vi "Main VI FTP FILE MANAGER.vi"() -> ()   [LabVIEW 2012]
doc: "FILE Archive & FTP is a software used to handle the file management of remote field sites using the HTI Data Logger or ATR series acoustic equipment that generates *.RAT and *.ATL files. The software monitors a specific folder on the local machine that the HTI equipment has been set up to move completed files of these types into. All other file types are ignored. The software continues to scan this file until a new file is added to the directory, on the addition of a file the NODE ARCHIVE & FTP software moves the file into an Archive directory (and if specified into a redundant Archive directory) then creates a *.ZIP version of the file and retains a copy of it in the Archive directory as well. All Zip files are then copied to a specified FTP host.\n\nNODE ARCHIVE & FTP will not try and move files for the last five minutes of an hour, or for the first five to ten minutes of the hour (based on CPU time). This is to allow the HTI hardware time to move all files at the top of the hour and avoid conflict. During the rest of the hour the software will continue to scan for new files. At any time a user can force a scan or FTP move by selecting the Manual Force FTP button or the Manual Archive Files button.\n\nNODE ARCHIVE & FTP creates an .INI file and a .CSV file in the programs application directory. The .INI file retains the last values of the file directory and FTP credentials used. The .CSV retains a history of *.ZIP files moved to the FTP and the status of their move, if there were errors or not. NODE ARCHIVE & FTP will continue to try and send the file to the FTP host until that file has completed the process with no errors. DO NOT remove or edit the .CSV file or the software will try and move all files up to the FTP again and will slow down the FTP Host."
uses:
  Controls/FTP Credintials.ctl
  Controls/File Management.ctl
  Controls/File Path directories.ctl
  Controls/Ping address and email notify.ctl
  Controls/PingElements.ctl
  SubVIs/Bini ArchiveAndFtpCluster.ctl
  <vilib>/Utility/sysdir.llb/System Directory Type.ctl
panel:
  in  "SaveConfig":bool
  in  "Settings":bool
  in  "Contacts":bool
  in  "Errors":bool
  in  "SetPingStats":bool
  in  "Addresses to Ping":T1
  in  "File type Cover":bool
  in  "Auto Archive":bool
  in  "Auto FTP":bool
  in  "update extentions":bool
  in  "ShutDown":bool
  in  "FTP Creds":T2={"Host"="", "UserName"="", "PassWord"="", "FTP File Path"="", "Timeout (S)"=0, "ActivePasive"=FALSE, "Binary Ascii"=FALSE, "Remote Port"=21} {"Timeout (S)" min=0 max=300 step=1}
  in  "SITE ID":string="Site Not Configured" caption="Site ID:"
  in  "File Management":T3
  in  "Manual FTP":bool
  out "Archive in progress":bool caption="Archive"
  out "Status FTP move":bool caption="FTP"
  in  "Manual Archive":bool
  in  "File output directories":T4={"Archive Location"=path "", "Archive Location 2"=path "<Not A Path>", "OutPut Path"=path "", "Directory(s) To Scan Files"=[]}
  in  "time date mod":bool
  out "Elapsed Time (H)":dbl caption="Time since Last File \nSize Check (H)" format="%#_3f"
  in  "recipients":string[](array[string])=["nmswyers@gmail.com"] caption="Errors & Warnings Email Recipients"
  out "hours":u8
  out "Email Notification Cluster":T5
  in  "shutting down closeout":bool
  in  "Time DaY":timestamp
  # "D\nI\nR\nE\nC\nT\nO\nR\nY\n\nS\nE\nT"
  # "FILE \n\nHANDLE\n\nMETHODS"
  # "FTP\n\nSETUP"
  # "Passive"
  # "Active"
  # "Binary"
  # "Ascii"
  # "File Handling Method"
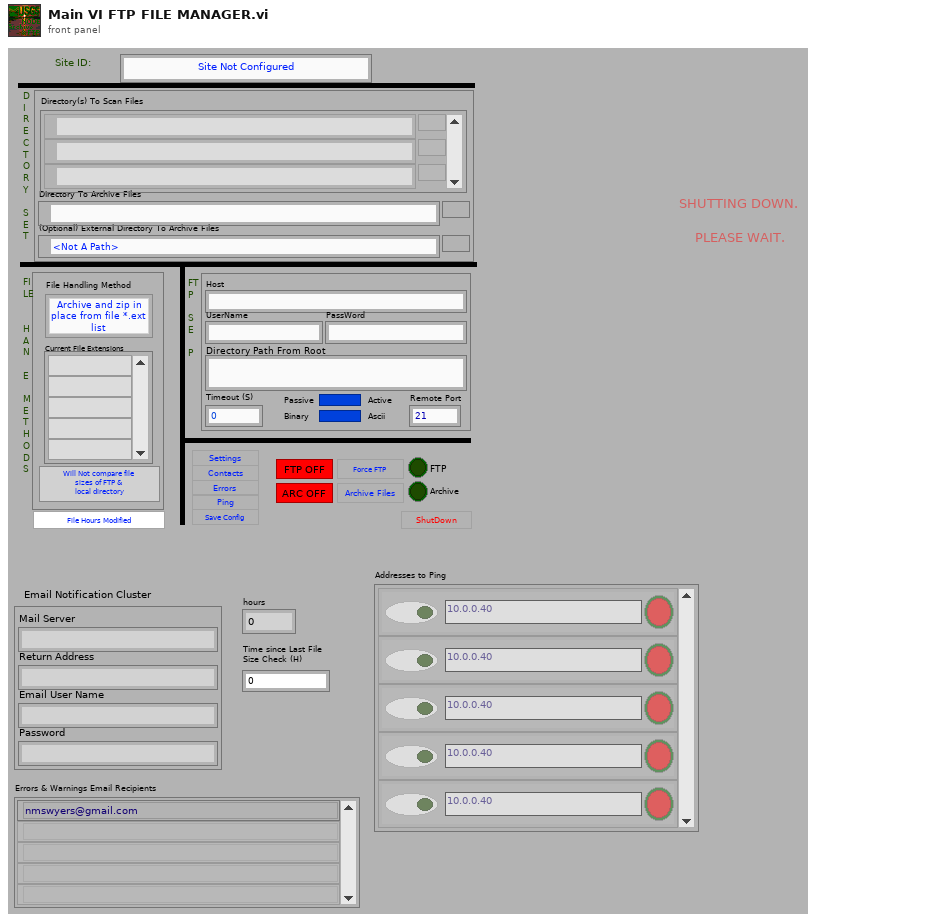
[diagram p1: front panel]
types:
  T1 = typedef "PingElements.ctl" = cluster{"AddressNode 1":string, "Response 1":bool, "Ping on Address 1":bool}[]
  T2 = typedef "FTP Credintials.ctl" = cluster{"Host":string, "UserName":string, "PassWord":string, "FTP File Path":string, "Timeout (S)":i32, "ActivePasive":bool, "Binary Ascii":bool, "Remote Port":u16}
  T3 = typedef "File Management.ctl" = cluster{"Comp File Size":bool, "File Handle Method":enum16{"Archive and zip in place from file *.ext list", "Archive and zip ALL file Types to archive directory", "Archive and zip to archive directory from file *.ext list", "Perform no file management"}, "file extention list":string[]}
  T4 = typedef "File Path directories.ctl" = cluster{"Archive Location":path, "Archive Location 2":path, "OutPut Path":path, "Directory(s) To Scan Files":path[]}
  T5 = typedef "Ping address and email notify.ctl" = cluster{"Mail Server":string, "Return Address":string, "Email User Name":string, "Password":string}
  T6 = enum16{"open", "replace", "create", "open or create", "replace or create", "replace or create with confirmation"}
  T7 = enum8{"Enabled", "Disabled", "Disabled and Grayed Out"}
  T8 = typedef "Bini ArchiveAndFtpCluster.ctl" = cluster{"Site ID":string, "File Management cluster":T3, "time stamp":timestamp, "File output directories":T4, "Auto FTP":bool, "Auto Archive":bool, "FTP CRED Cluster":T2, "hours old date mod(hours)":u8, "Email Notification Cluster":T5, "Email Recipiant List":string[], "Addresses to Ping":T1}
  T9 = enum16{"Archive and zip in place from file *.ext list", "Archive and zip ALL file Types to archive directory", "Archive and zip to archive directory from file *.ext list", "Perform no file management"}
  T10 = enum32{"Invalid", "Standard", "Closed", "Hidden", "Minimized", "Maximized"}
  T11 = cluster{"AddressNode 1":string, "Response 1":bool, "Ping on Address 1":bool}
  T12 = enum32{"invalid app kind", "Development System", "Run Time System", "Student Edition", "Embedded LabVIEW", "Evaluation", "Custom"}
  T13 = typedef "System Directory Type.ctl" = i32
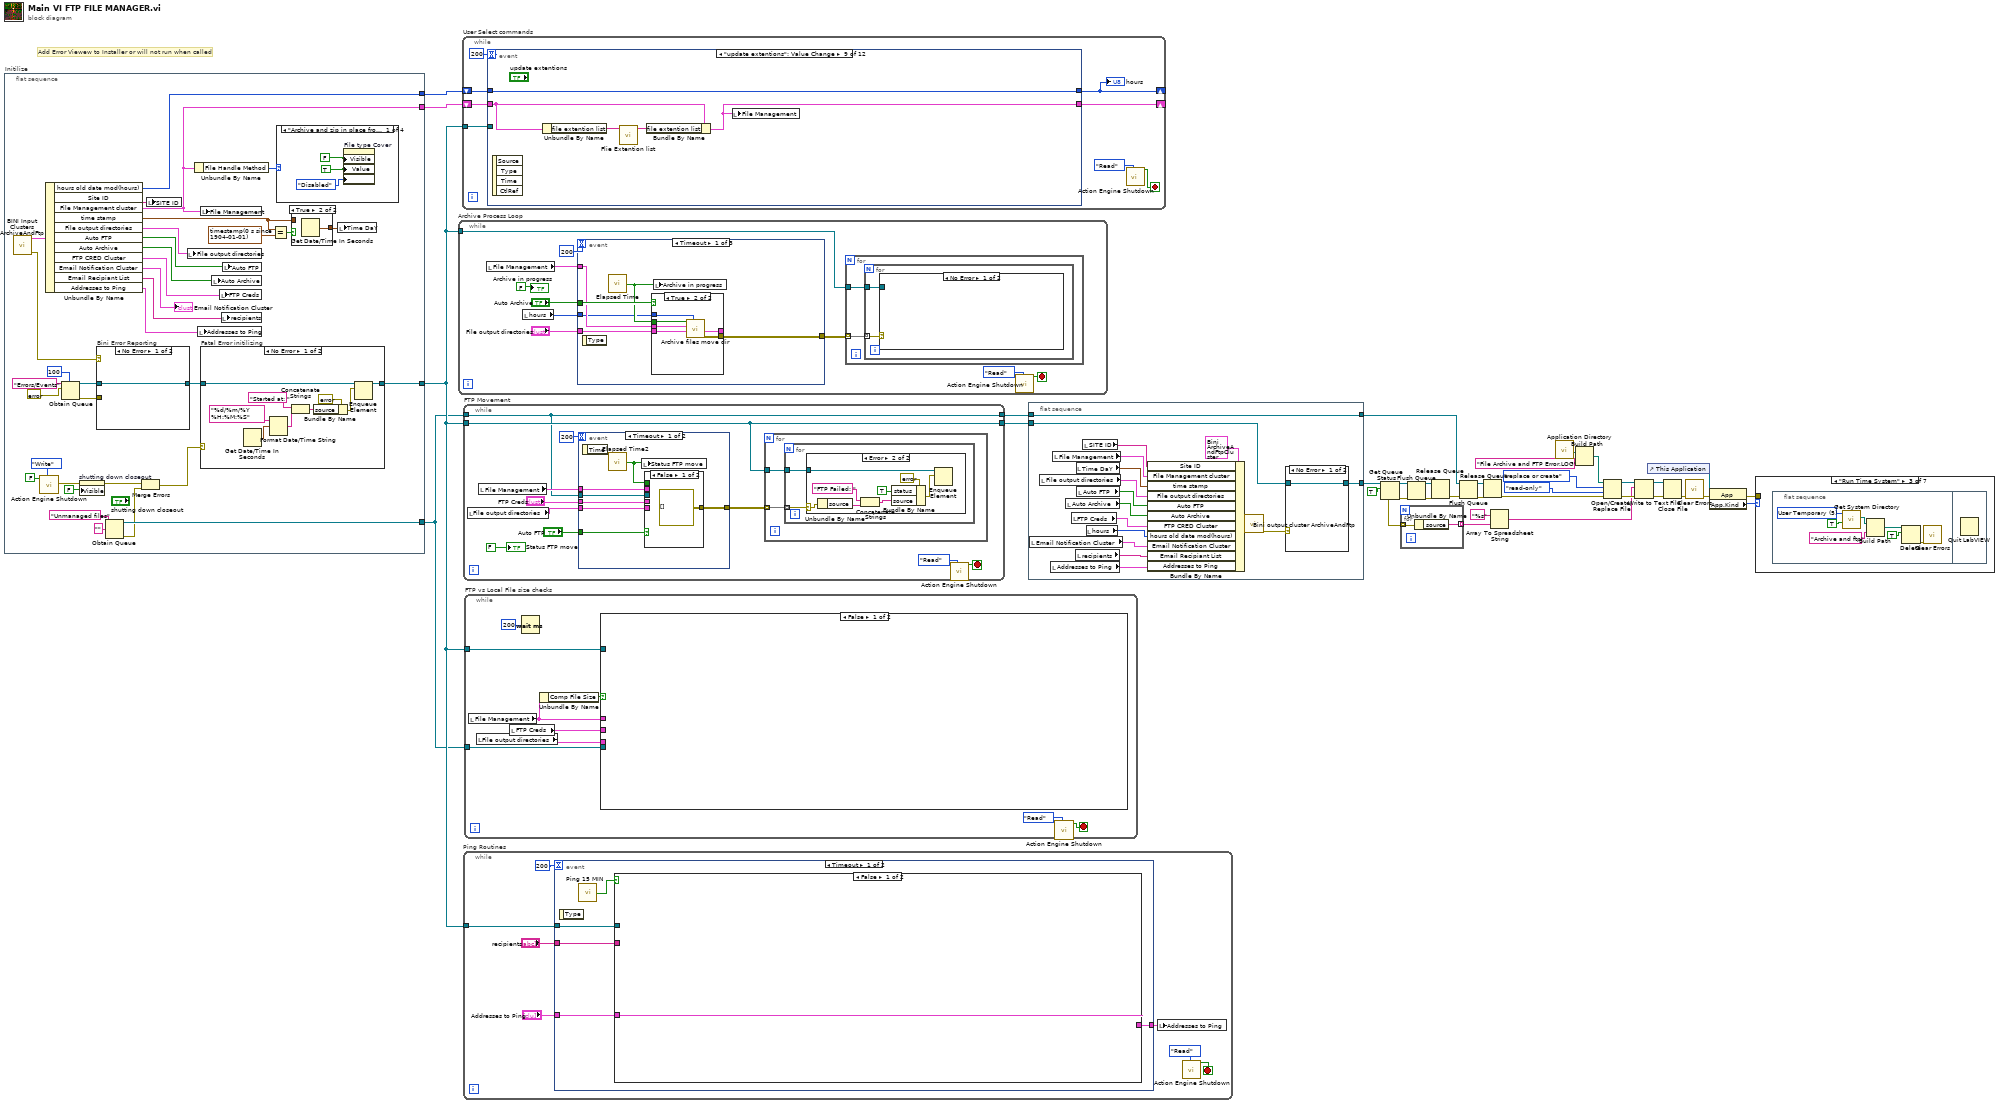
[diagram p0: block diagram]
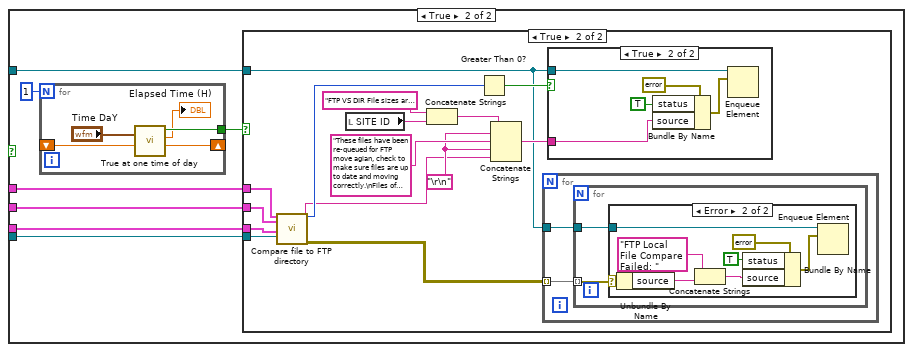
[diagram p2: hidden frame]
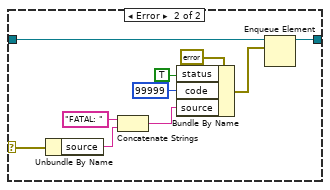
[diagram p7: hidden frame]
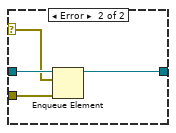
[diagram p8: hidden frame]
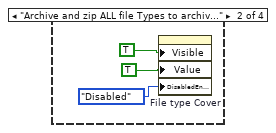
[diagram p9: hidden frame]
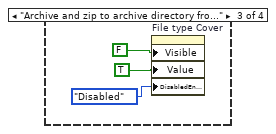
[diagram p10: hidden frame]
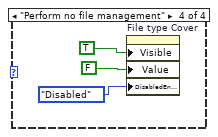
[diagram p11: hidden frame]
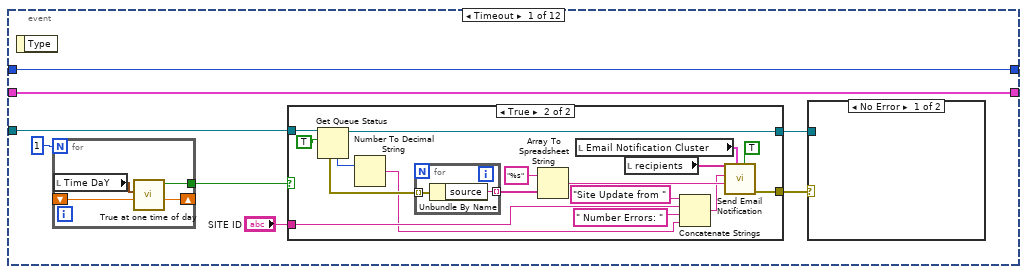
[diagram p12: hidden frame]
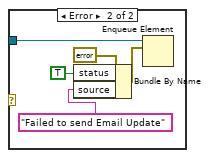
[diagram p13: hidden frame]
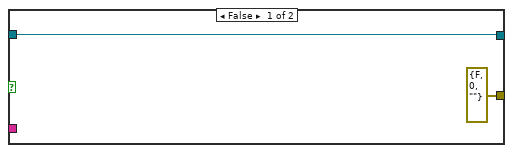
[diagram p14: hidden frame]
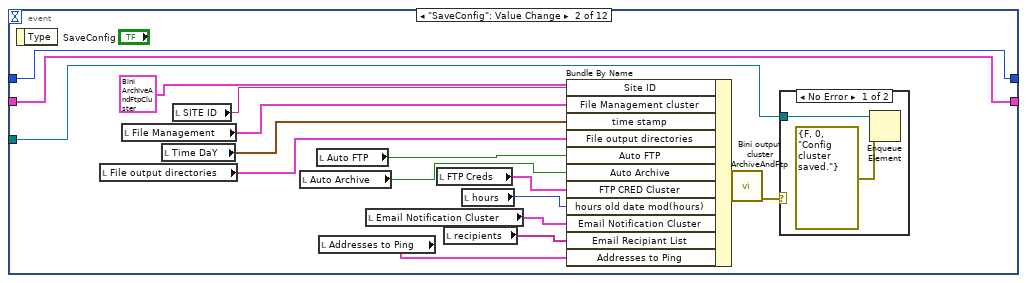
[diagram p15: hidden frame]
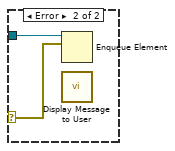
[diagram p16: hidden frame]
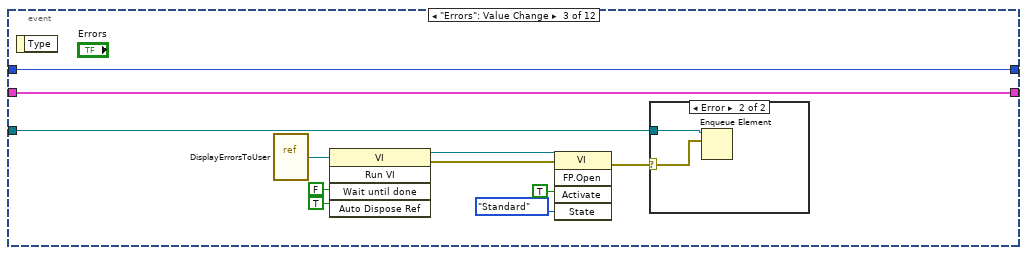
[diagram p17: hidden frame]
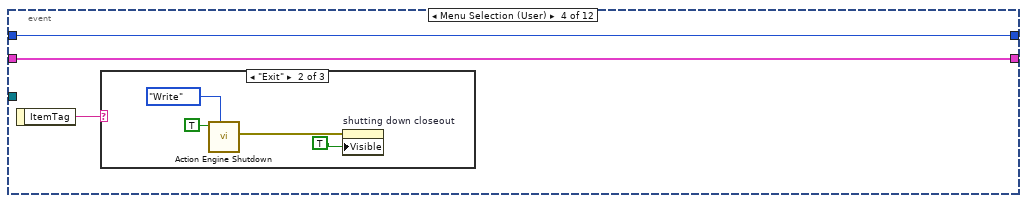
[diagram p19: hidden frame]
diagram:
  # "Add Error Viewew to Installer or will not run when called"
  n1 = flat-sequence "Initilize" {
    tunnel: [w67] -> w29
    tunnel: [w57] -> w32
    tunnel: [w52] -> w31
    tunnel: [w40] -> w30
    frame #0 {
      n2 = call "BINI Input Clusters ArchiveAndFtp.vi"() -> ("Bini Error out"=w47:errorcluster, "Bini Load"=w58:T8)  [unwired: 10 in]
      n3 = call "Action Engine Shutdown.vi"("Shutdown"=enum16{"Write", "Read"}."Write", "Shutdown (True to Shutdown)"=FALSE) -> ("error out"=w63:errorcluster)  [unwired: 8 in, 1 out]
      n4 = Unbundle By Name(w58) -> ("hours old date mod(hours)"=w52:u8, "Site ID"=w56:string, "File Management cluster"=w57:T3, "time stamp"=w36:timestamp, "File output directories"=w55:T4, "Auto FTP"=w54:bool, "Auto Archive"=w53:bool, "FTP CRED Cluster"=w51:T2, "Email Notification Cluster"=→"Email Notification Cluster":T5, "Email Recipiant List"=w49:string[], "Addresses to Ping"=w48:T1)
      n5 = Obtain Queue(max queue size (-1, unlimited)=100, name (unnamed)="Errors/Events", element data type=errorcluster {"status"=FALSE, "code"=0, "source"=""} ("error constant")) -> (queue out=w46:refnum<queue>, error out=w44:errorcluster)  [unwired: 2 in, 1 out]
      n6 = property on="shutting down closeout" class="Bool"(error in=w63, "Visible"=FALSE) -> (error out=w43:errorcluster)  [unwired: 1 in, 1 out]
      n7 = case "Bini Error Reporting" shown="No Error" w47 {
        selector: w47 -> [_ w93]
        tunnel: w46 -> [w91 w95]
        tunnel: [w91 w94] -> w41
        tunnel: w44 -> [_ w92]
        frame No Error {
        }
        frame Error {
          n8 = Enqueue Element(queue=w95, element=w93, error in (no error)=w92) -> (queue out=w94:refnum<queue>)  [unwired: 1 in, 2 out]
        }
      }
      n9 = Obtain Queue(name (unnamed)="Unmanaged files", element data type="" ("name (unnamed)")) -> (queue out=w67:refnum<queue>, error out=w61:errorcluster)  [unwired: 3 in, 1 out]
      n10 = Merge Errors(w43, w61) -> (w42:errorcluster)
      n11 = local write "SITE ID"(w56) -> ()
      n12 = local write "File output directories"(w55) -> ()
      n13 = Unbundle By Name(w57) -> ("File Handle Method"=w62:T9)
      n14 = local write "Addresses to Ping"(w48) -> ()
      n15 = local write "File Management"(w57) -> ()
      n16 = case "Fatal Error initilizing" shown="No Error" w42 {
        selector: w42 -> [_ w84]
        tunnel: w41 -> [w80 w90]
        tunnel: [w79 w89] -> w40
        frame No Error {
          n17 = Get Date/Time In Seconds() -> (seconds since 1Jan1904=w74:timestamp)
          n18 = Format Date/Time String(time format string (%c)="%d/%m/%Y %H:%M:%S", seconds (now)=w74) -> (date/time string=w73:string)  [unwired: 1 in]
          n19 = Concatenate Strings("Started at: " ("string"), w73) -> (w76:string)
          n20 = Bundle By Name(cluster=errorcluster {"status"=FALSE, "code"=0, "source"=""} ("element"), "source"=w76) -> (w77:errorcluster)
          n21 = Enqueue Element(queue=w80, element=w77) -> (queue out=w79:refnum<queue>)  [unwired: 2 in, 2 out]
        }
        frame Error {
          n22 = Unbundle By Name(w84) -> ("source"=w83:string)
          n23 = Concatenate Strings("FATAL: " ("string"), w83) -> (w86:string)
          n24 = Bundle By Name(cluster=errorcluster {"status"=FALSE, "code"=0, "source"=""} ("error constant"), "status"=TRUE, "code"=99999, "source"=w86) -> (w81:errorcluster)
          n25 = Enqueue Element(queue=w90, element=w81) -> (queue out=w89:refnum<queue>)  [unwired: 2 in, 2 out]
        }
      }
      n26 = local write "Auto Archive"(w53) -> ()
      n27 = local write "FTP Creds"(w51) -> ()
      n28 = local write "recipients"(w49) -> ()
      n29 = local write "Auto FTP"(w54) -> ()
      n30 = Equal?(x=w36, y=timestamp(0 s since 1904-01-01)) -> (x = y?=w39:bool)
      n31 = case shown="\"Archive and zip in place from file *.ext list\", Default" w62 {
        frame "Archive and zip in place from file *.ext list", Default {
          n32 = property on="File type Cover" class="Bool (strict)"("Visible"=FALSE, "Value"=TRUE ("File type Cover"), "DisabledEnum"=T7."Disabled" ("Disabled")) -> ()  [unwired: 2 in, 2 out]
        }
        frame "Archive and zip ALL file Types to archive directory" {
          n33 = property on="File type Cover" class="Bool (strict)"("Visible"=TRUE, "Value"=TRUE ("File type Cover"), "DisabledEnum"=T7."Disabled" ("Disabled")) -> ()  [unwired: 2 in, 2 out]
        }
        frame "Archive and zip to archive directory from file *.ext list" {
          n34 = property on="File type Cover" class="Bool (strict)"("Visible"=FALSE, "Value"=TRUE ("File type Cover"), "DisabledEnum"=T7."Disabled" ("Disabled")) -> ()  [unwired: 2 in, 2 out]
        }
        frame "Perform no file management" {
          n35 = property on="File type Cover" class="Bool (strict)"("Visible"=TRUE, "Value"=FALSE ("File type Cover"), "DisabledEnum"=T7."Disabled" ("Disabled")) -> ()  [unwired: 2 in, 2 out]
        }
      }
      n36 = case shown="True" w39 {
        tunnel: [w70 w71] -> w37
        tunnel: w36 -> [w70 _]
        frame False {
        }
        frame True {
          n37 = Get Date/Time In Seconds() -> (seconds since 1Jan1904=w71:timestamp)
        }
      }
      n38 = local write "Time DaY"(w37) -> ()
    }
  }
  n39 = while "Archive Process Loop" {
    tunnel: w30 -> [w109]
    stop <- w113 stop-if-true
    n40 = local read "File Management"() -> (w108:T3)
    n41 = local read "hours"() -> (w110:u8)
    n42 = event shown="[0] Timeout" {
      selector: _ -> [_ _ _]
      dyn-events: _ -> [_ _ _]
      timeout: 200 -> [_ _ _]
      tunnel: [w135 w148 errorcluster[][] [] ("ErrorArray")] -> w112
      tunnel: "File output directories" -> [w130 w147 _]
      tunnel: w108 -> [w133 w145 _]
      tunnel: "Auto Archive" -> [w134 _ _]
      tunnel: w110 -> [w131 w144 _]
      event Timeout {
        n43 = event-data() -> ()  [unwired: 1 in, 1 out]
        n44 = call "Elapsed Time"() -> ("Time has Elapsed"=w132:bool)  [unwired: 12 in, 7 out]
        n45 = case shown="True" w134 {
          tunnel: w130 -> [w137 w143]
          tunnel: [errorcluster[][] [] ("ErrorArray") w142] -> w135
          tunnel: w133 -> [_ w141]
          tunnel: w132 -> [_ w140]
          tunnel: w131 -> [_ w139]
          tunnel: [w137 w138] -> _
          frame False {
          }
          frame True {
            n46 = call "Archive files move dir.vi"("hours old date mod(hours)"=w139, "File path input cluster"=w143, "File Management"=w141, "Timing True to archive"=w140) -> ("ErrorArray"=w142:errorcluster[][], "File path input cluster (out)"=w138:T4)  [unwired: 4 in]
          }
        }
        n47 = local write "Archive in progress"(w132) -> ()
      }
      event "Manual Archive": Value Change {
        w146 = TRUE ("Status File move")
        n48 = event-data() -> ()  [unwired: 1 in, 1 out]
        n49 = local write "Archive in progress"(w146) -> ()
        n50 = call "Archive files move dir.vi"("hours old date mod(hours)"=w144, "File path input cluster"=w147, "File Management"=w145, "Timing True to archive"=w146) -> ("ErrorArray"=w148:errorcluster[][])  [unwired: 4 in, 1 out]
      }
      event Value Change {
        n51 = event-data() -> ("NewVal"=w150:T9)  [unwired: 1 in]
        n52 = case shown="\"Archive and zip ALL file Types to archive directory\"" w150 {
          frame "Archive and zip in place from file *.ext list", Default {
            n53 = property on="File type Cover" class="Bool (strict)"("Visible"=FALSE, "Value"=TRUE ("File type Cover"), "DisabledEnum"=T7."Disabled" ("Disabled")) -> ()  [unwired: 2 in, 2 out]
          }
          frame "Archive and zip ALL file Types to archive directory" {
            n54 = property on="File type Cover" class="Bool (strict)"("Visible"=TRUE, "Value"=TRUE ("File type Cover"), "DisabledEnum"=T7."Disabled" ("Disabled")) -> ()  [unwired: 2 in, 2 out]
          }
          frame "Archive and zip to archive directory from file *.ext list" {
            n55 = property on="File type Cover" class="Bool (strict)"("Visible"=FALSE, "Value"=TRUE ("File type Cover"), "DisabledEnum"=T7."Disabled" ("Disabled")) -> ()  [unwired: 2 in, 2 out]
          }
          frame "Perform no file management" {
            n56 = property on="File type Cover" class="Bool (strict)"("Visible"=TRUE, "Value"=FALSE ("File type Cover"), "DisabledEnum"=T7."Disabled" ("Disabled")) -> ()  [unwired: 2 in, 2 out]
          }
        }
      }
    }
    n57 = for {
      tunnel: w112 -> [w119] mode=indexing
      tunnel: w109 -> [w118]
      n58 = for {
        tunnel: w119 -> [w121] mode=indexing
        tunnel: w118 -> [w120]
        n59 = case shown="No Error" w121 {
          selector: w121 -> [_ w124]
          tunnel: w120 -> [_ w129]
          frame No Error {
          }
          frame Error {
            n60 = Unbundle By Name(w124) -> ("source"=w123:string)
            n61 = Concatenate Strings("Archiving Process: " ("string"), w123) -> (w122:string)
            n62 = Bundle By Name(cluster=errorcluster {"status"=FALSE, "code"=0, "source"=""} ("error constant"), "status"=TRUE, "source"=w122) -> (w127:errorcluster)
            n63 = Enqueue Element(queue=w129, element=w127) -> ()  [unwired: 2 in, 3 out]
          }
        }
      }
    }
    n64 = call "Action Engine Shutdown.vi"("Shutdown"=enum16{"Write", "Read"}."Read") -> ("Shutdown"=w113:bool)  [unwired: 9 in, 1 out]
    "Archive in progress" <- FALSE ("Archive in progress")
  }
  n65 = while "User Select commands" {
    shift-right: [w166] -> _
    shift-left: w31 -> [w167]
    shift-right: [w164] -> _
    shift-left: w32 -> [w165]
    tunnel: w30 -> [w163]
    stop <- w168 stop-if-true
    n66 = event shown="[8] \"update extentions\": Value Change" {
      selector: _ -> [_ _ _ _ _ _ _ _ _ _ _ _]
      dyn-events: _ -> [_ _ _ _ _ _ _ _ _ _ _ _]
      timeout: 200 -> [_ _ _ _ _ _ _ _ _ _ _ _]
      tunnel: w167 -> [w178 w212 w240 w244 w251 w259 w265 w272 w290 w296 w300 w304]
      tunnel: [w178 w212 w240 w244 w251 w259 w265 w271 w290 w296 w300 w304] -> w166
      tunnel: w165 -> [w177 w211 w239 w243 w250 w258 w264 w270 w293 _ w299 w303]
      tunnel: [w177 w211 w239 w243 w250 w258 w264 w270 w291 "File Management" w299 w303] -> w164
      tunnel: w163 -> [w173 w209 w230 _ _ _ _ _ _ _ _ _]
      event Timeout {
        n67 = event-data() -> ()  [unwired: 1 in, 1 out]
        n68 = for {
          N: 1 -> [_]
          tunnel: [w208] -> w176
          shift-right: [w207] -> _
          shift-left: _ -> [w206]
          n69 = local read "Time DaY"() -> (w205:timestamp)
          n70 = call "True at one time of day.vi"("Next start time in"=w206, "Time stamp from INI (only will use time Not date)"=w205) -> ("next start time out"=w207:dbl, "Time has Elapsed"=w208:bool)  [unwired: 6 in, 2 out]
        }
        n71 = case shown="True" w176 {
          tunnel: "SITE ID" -> [_ w190]
          tunnel: w173 -> [w184 w198]
          tunnel: [errorcluster {"status"=FALSE, "code"=0, "source"=""} ("error out") w199] -> w172
          tunnel: [w184 w186] -> w171
          frame False {
          }
          frame True {
            n72 = Get Queue Status(queue=w198, return elements? (F)=TRUE) -> (queue out=w186:refnum<queue>, # elements in queue=w189:i32, elements=w196:errorcluster[])  [unwired: 1 in, 5 out]
            n73 = Number To Decimal String(number=w189) -> (decimal integer string=w187:string)  [unwired: 1 in]
            n74 = for {
              tunnel: w196 -> [w204] mode=indexing
              tunnel: [w203] -> w195 mode=indexing
              n75 = Unbundle By Name(w204) -> ("source"=w203:string)
            }
            n76 = Array To Spreadsheet String(array=w195, 3:"%s" ("format string")) -> (spreadsheet string=w193:string)  [unwired: 1 in]
            n77 = local read "Email Notification Cluster"() -> (w200:T5)
            n78 = local read "recipients"() -> (w202:string[])
            n79 = Concatenate Strings("Site Update from " ("string"), w190, " Number Errors: " ("string"), w187) -> (w192:string)
            n80 = call "Send Email Notification.vi"("Send Email Notification"=TRUE, "Email Notification Cluster (in)"=w200, "message"=w193, "Email Subject"=w192, "recipients"=w202) -> ("error out"=w199:errorcluster)  [unwired: 6 in]
          }
        }
        n81 = case shown="No Error" w172 {
          tunnel: w171 -> [_ w183]
          frame No Error {
          }
          frame Error {
            n82 = Bundle By Name(cluster=errorcluster {"status"=FALSE, "code"=0, "source"=""} ("error constant"), "status"=TRUE, "source"="Failed to send Email Update") -> (w181:errorcluster)
            n83 = Enqueue Element(queue=w183, element=w181) -> ()  [unwired: 2 in, 3 out]
          }
        }
      }
      event "SaveConfig": Value Change {
        n84 = event-data() -> ()  [unwired: 1 in, 1 out]
        n85 = local read "File output directories"() -> (w218:T4)
        n86 = local read "File Management"() -> (w216:T3)
        n87 = local read "Time DaY"() -> (w217:timestamp)
        n88 = local read "SITE ID"() -> (w215:string)
        n89 = local read "Auto Archive"() -> (w220:bool)
        n90 = local read "Auto FTP"() -> (w219:bool)
        n91 = local read "Addresses to Ping"() -> (w225:T1)
        n92 = local read "Email Notification Cluster"() -> (w223:T5)
        n93 = local read "FTP Creds"() -> (w221:T2)
        n94 = local read "recipients"() -> (w224:string[])
        n95 = local read "hours"() -> (w222:u8)
        n96 = Bundle By Name(cluster=T8 {"Site ID"="", "File Management cluster"={"Comp File Size"=FALSE, "File Handle Method"=enum."Archive and zip in place from file *.ext list", "file extention list"=[]}, "time stamp"=timestamp(0 s since 1904-01-01), "File output directories"={"Archive Location"=path "", "Archive Location 2"=path "<Not A Path>", "OutPut Path"=path "", "Directory(s) To Scan Files"=[]}, "Auto FTP"=FALSE, "Auto Archive"=FALSE, "FTP CRED Cluster"={"Host"="", "UserName"="", "PassWord"="", "FTP File Path"="", "Timeout (S)"=60, "ActivePasive"=FALSE, "Binary Ascii"=FALSE, "Remote Port"=0}, "hours old date mod(hours)"=2, "Email Notification Cluster"={"Mail Server"="", "Return Address"="", "Email User Name"="", "Password"=""}, "Email Recipiant List"=[], "Addresses to Ping"=[]} ("Settings To Bini"), "Site ID"=w215, "File Management cluster"=w216, "time stamp"=w217, "File output directories"=w218, "Auto FTP"=w219, "Auto Archive"=w220, "FTP CRED Cluster"=w221, "hours old date mod(hours)"=w222, "Email Notification Cluster"=w223, "Email Recipiant List"=w224, "Addresses to Ping"=w225) -> (w214:T8)
        n97 = call "Bini output cluster ArchiveAndFtp.vi"("Settings To Bini"=w214) -> ("Bini Error out"=w210:errorcluster)  [unwired: 14 in]
        n98 = case shown="No Error" w210 {
          selector: w210 -> [_ w228]
          tunnel: w209 -> [w227 w229]
          frame No Error {
            n99 = Enqueue Element(queue=w227, element=errorcluster {"status"=FALSE, "code"=0, "source"="Config cluster saved."}) -> ()  [unwired: 2 in, 3 out]
          }
          frame Error {
            n100 = Enqueue Element(queue=w229, element=w228) -> ()  [unwired: 2 in, 3 out]
            n101 = call "Display Message to User"() -> ()  [unwired: 10 in, 2 out]
          }
        }
      }
      event "Errors": Value Change {
        n102 = event-data() -> ()  [unwired: 1 in, 1 out]
        n103 = vi-ref "DisplayErrorsToUser.vi"() -> (w238:refnum<vi>)
        n104 = invoke class="VI" method="Run VI"(reference=w238, "Wait until done"=FALSE ("Wait Until Done"), "Auto Dispose Ref"=TRUE ("Auto Dispose Reference")) -> (reference out=w235:refnum<vi>, error out=w234:errorcluster)  [unwired: 2 in, 3 out]
        n105 = invoke class="VI" method="FP.Open"(reference=w235, error in=w234, "Activate"=TRUE ("Activate?"), "State"=T10."Standard") -> (error out=w231:errorcluster)  [unwired: 1 in, 4 out]
        n106 = case shown="Error" w231 {
          selector: w231 -> [_ w241]
          tunnel: w230 -> [_ w242]
          frame No Error {
          }
          frame Error {
            n107 = Enqueue Element(queue=w242, element=w241) -> ()  [unwired: 2 in, 3 out]
          }
        }
      }
      event Menu Selection (User) {
        n108 = event-data() -> ("ItemTag"=w245:string)  [unwired: 1 in]
        n109 = case shown="\"Exit\"" w245 {
          frame "Null", Default {
          }
          frame "Exit" {
            n110 = call "Action Engine Shutdown.vi"("Shutdown"=enum16{"Write", "Read"}."Write", "Shutdown (True to Shutdown)"=TRUE ("Stop Button")) -> ("error out"=w246:errorcluster)  [unwired: 8 in, 1 out]
            n111 = property on="shutting down closeout" class="Bool"(error in=w246, "Visible"=TRUE) -> ()  [unwired: 1 in, 2 out]
          }
          frame "NAF" {
            n112 = call "About.vi"() -> ()  [unwired: 12 in]
          }
        }
      }
      event "ShutDown": Value Change {
        n113 = event-data() -> ()  [unwired: 1 in, 1 out]
        n114 = Two Button Dialog(message="Are you sure you want to shut down the software? This will end all file management of the Archive directories and FTP file movement until the software is restarted.\nIf the Archiving In Progress, or the FTP In Progress is lit the software will shut down as soon as the process is done.", 2:"Shutdown" ("T button name (\"OK\")")) -> (T button?=w254:bool)  [unwired: 1 in]
        n115 = case shown="True" w254 {
          frame False {
          }
          frame True {
            n116 = property on="shutting down closeout" class="Bool"("Visible"=TRUE) -> ()  [unwired: 2 in, 2 out]
            n117 = call "Action Engine Shutdown.vi"("Shutdown"=enum16{"Write", "Read"}."Write", "Shutdown (True to Shutdown)"=TRUE) -> ()  [unwired: 8 in, 2 out]
          }
        }
      }
      event Application Instance Close? {
        w263 = TRUE ("SilentShutdown")
        n118 = event-data() -> ()  [unwired: 1 in, 1 out]
        n119 = call "Action Engine Shutdown.vi"("Shutdown"=enum16{"Write", "Read"}."Write", "Shutdown (True to Shutdown)"=TRUE) -> ()  [unwired: 8 in, 2 out]
        n120 = property on="shutting down closeout" class="Bool"("Visible"=TRUE) -> ()  [unwired: 2 in, 2 out]
        n121 = event-data("SilentShutdown"=w263, "Discard?"=w263) -> ()  [unwired: 1 in, 1 out]
      }
      event Panel Close? {
        n122 = event-data() -> ()  [unwired: 1 in, 1 out]
        n123 = call "Action Engine Shutdown.vi"("Shutdown"=enum16{"Write", "Read"}."Write", "Shutdown (True to Shutdown)"=TRUE) -> ()  [unwired: 8 in, 2 out]
        n124 = property on="shutting down closeout" class="Bool"("Visible"=TRUE) -> ()  [unwired: 2 in, 2 out]
        n125 = event-data("Discard?"=TRUE) -> ()  [unwired: 1 in, 1 out]
      }
      event "time date mod": Value Change {
        n126 = event-data() -> ()  [unwired: 1 in, 1 out]
        n127 = Number To Decimal String(number=w272) -> (decimal integer string=w280:string)  [unwired: 1 in]
        n128 = Concatenate Strings("The Current number of hours that need to passed on a files last modified date before the file will be archived and moved to the ftp server." ("Message"), "\r\n", w280) -> (w278:string)
        n129 = call "Display Message to User2"("Message"=w278) -> ("error out"=w275:errorcluster, "Change Value"=w276:bool)  [unwired: 9 in]
        n130 = call "Prompt User for Input2"("Enable"=w276, "error in (no error)"=w275) -> ("(Hours)"=w274:dbl, "OK"=w273:bool, "error out"=w281:errorcluster)  [unwired: 15 in]
        n131 = case shown="No Error" w281 {
          tunnel: w273 -> [w285 _]
          tunnel: w274 -> [w284 _]
          tunnel: [w283 w289] -> w271
          tunnel: w272 -> [w282 w289]
          frame No Error {
            n132 = case shown="True" w285 {
              tunnel: w284 -> [_ w288]
              tunnel: w282 -> [w286 _]
              tunnel: [w286 w287] -> w283
              frame False {
              }
              frame True {
                n133 = To Unsigned Byte Integer(number=w288) -> (unsigned 8bit integer=w287:u8)
              }
            }
          }
          frame Error {
          }
        }
      }
      event "update extentions": Value Change {
        n134 = event-data() -> ()  [unwired: 1 in, 4 out]
        n135 = Unbundle By Name(w293) -> ("file extention list"=w292:string[])
        n136 = call "Flie Extention list.vi"("file extention list IN"=w292) -> ("File extention list (out)"=w294:string[])  [unwired: 10 in]
        n137 = Bundle By Name(cluster=w293, "file extention list"=w294) -> (w291:T3)
        n138 = local write "File Management"(w291) -> ()
      }
      event Value Change {
        n139 = event-data() -> ()  [unwired: 1 in, 4 out]
        n140 = local write "File Management"("File Management") -> ()
      }
      event "Contacts": Value Change {
        n141 = event-data() -> ()  [unwired: 1 in, 1 out]
        n142 = local read "recipients"() -> (w298:string[])
        n143 = call "SetContactList.vi"("recipients IN"=w298) -> ("recipients OUT"=w297:string[])  [unwired: 10 in]
        n144 = local write "recipients"(w297) -> ()
      }
      event "Settings": Value Change {
        n145 = event-data() -> ()  [unwired: 1 in, 1 out]
        n146 = local read "Email Notification Cluster"() -> (w302:T5)
        n147 = call "GeneralSettingsConfigure.vi"("Email Notification Cluster in"=w302) -> ("Email Notification Cluster out"=w301:T5)  [unwired: 10 in]
        n148 = local write "Email Notification Cluster"(w301) -> ()
      }
    }
    "hours" <- w166
    n149 = call "Action Engine Shutdown.vi"("Shutdown"=enum16{"Write", "Read"}."Read") -> ("Shutdown"=w168:bool)  [unwired: 9 in, 1 out]
  }
  n150 = while "Ping Routines" {
    tunnel: w30 -> [w307]
    stop <- w308 stop-if-true
    n151 = event shown="[0] Timeout" {
      selector: _ -> [_ _]
      dyn-events: _ -> [_ _]
      timeout: 200 -> [_ _]
      tunnel: "recipients" -> [w315 _]
      tunnel: "Addresses to Ping" -> [w314 w374]
      tunnel: w307 -> [w313 _]
      tunnel: [w312 w373] -> w306
      event Timeout {
        n152 = event-data() -> ()  [unwired: 1 in, 1 out]
        n153 = call "Ping 15 MIN"() -> ("Time has Elapsed"=w316:bool)  [unwired: 12 in, 7 out]
        n154 = case shown="False" w316 {
          tunnel: w315 -> [_ w321]
          tunnel: w314 -> [w317 w320]
          tunnel: w313 -> [_ w319]
          tunnel: [w317 w318] -> w312
          frame False {
          }
          frame True {
            n155 = for {
              tunnel: w321 -> [w329]
              tunnel: w320 -> [w324] mode=indexing
              tunnel: w319 -> [w323]
              tunnel: [w322] -> w318 mode=indexing
              stop <- w326 stop-if-true
              n156 = Unbundle By Name(w324) -> ("AddressNode 1"=w325:string, "Ping on Address 1"=w328:bool)
              n157 = case shown="True" w328 {
                tunnel: w325 -> [_ w337]
                tunnel: w329 -> [_ w340]
                tunnel: w324 -> [w332 w338]
                tunnel: w323 -> [_ w334]
                tunnel: [w330 w333] -> w322
                frame False {
                  n158 = Bundle By Name(cluster=w332, "Response 1"=FALSE) -> (w330:T11)
                }
                frame True {
                  n159 = call "Online Status through Ping.vi"("AddressToPing"=w337, "Ping Method"=enum16{"LongPing", "NormalPing", "FastPing"}."FastPing") -> ("Connection?"=w339:bool, "error out"=w335:errorcluster)  [unwired: 9 in, 3 out]
                  n160 = case shown="No Error" w335 {
                    selector: w335 -> [_ w365]
                    tunnel: w340 -> [w346 _]
                    tunnel: w339 -> [w345 _]
                    tunnel: w338 -> [w344 w368]
                    tunnel: w337 -> [w343 w362]
                    tunnel: w334 -> [w342 w372]
                    tunnel: [w341 w366] -> w333
                    frame No Error {
                      n161 = case shown="False" w345 {
                        tunnel: w346 -> [_ _]
                        tunnel: w343 -> [w347 _]
                        tunnel: w344 -> [w356 w359]
                        tunnel: w342 -> [w353 _]
                        tunnel: [w355 w357] -> w341
                        frame False {
                          n162 = Bundle By Name(cluster=w356, "Response 1"=FALSE) -> (w355:T11)
                          n163 = Concatenate Strings("Unable to Ping: " ("string"), w347) -> (w349:string)
                          n164 = Bundle By Name(cluster=errorcluster {"status"=FALSE, "code"=0, "source"=""} ("error constant"), "status"=FALSE, "source"=w349) -> (w351:errorcluster)
                          n165 = Enqueue Element(queue=w353, element=w351) -> ()  [unwired: 2 in, 3 out]
                        }
                        frame True {
                          n166 = Bundle By Name(cluster=w359, "Response 1"=TRUE) -> (w357:T11)
                        }
                      }
                    }
                    frame Error {
                      n167 = Unbundle By Name(w365) -> ("source"=w360:string)
                      n168 = Bundle By Name(cluster=w368, "Response 1"=FALSE) -> (w366:T11)
                      n169 = Concatenate Strings("Ping Request Failed on IP: " ("string"), w362, " : " ("string"), w360) -> (w364:string)
                      n170 = Bundle By Name(cluster=errorcluster {"status"=FALSE, "code"=0, "source"=""} ("error constant"), "status"=TRUE, "source"=w364) -> (w370:errorcluster)
                      n171 = Enqueue Element(queue=w372, element=w370) -> ()  [unwired: 2 in, 3 out]
                    }
                  }
                }
              }
              n172 = call "Action Engine Shutdown.vi"("Shutdown"=enum16{"Write", "Read"}."Read") -> ("Shutdown"=w326:bool)  [unwired: 9 in, 1 out]
            }
          }
        }
      }
      event "SetPingStats": Value Change {
        n173 = event-data() -> ()  [unwired: 1 in, 1 out]
        n174 = call "SetPingAddresses.vi"("Addresses to Ping(in)"=w374) -> ("Addresses to Ping(out)"=w373:T1)  [unwired: 10 in]
      }
    }
    n175 = local write "Addresses to Ping"(w306) -> ()
    n176 = call "Action Engine Shutdown.vi"("Shutdown"=enum16{"Write", "Read"}."Read") -> ("Shutdown"=w308:bool)  [unwired: 9 in, 1 out]
  }
  n177 = while "FTP Movement" {
    tunnel: w29 -> [w376]
    tunnel: w30 -> [w377]
    tunnel: [w377] -> w28
    tunnel: [w376] -> w7
    stop <- w379 stop-if-true
    n178 = local read "File output directories"() -> (w383:T4)
    n179 = local read "File Management"() -> (w381:T3)
    n180 = event shown="[0] Timeout" {
      selector: _ -> [_ _]
      dyn-events: _ -> [_ _]
      timeout: 200 -> [_ _]
      tunnel: w376 -> [w404 w415]
      tunnel: [w403 w416] -> w375
      tunnel: "FTP Creds" -> [w402 w414]
      tunnel: w383 -> [w400 w412]
      tunnel: w381 -> [w401 w413]
      tunnel: "Auto FTP" -> [w399 _]
      event Timeout {
        n181 = event-data() -> ()  [unwired: 1 in, 1 out]
        n182 = call "Elapsed Time2"() -> ("Time has Elapsed"=w398:bool)  [unwired: 12 in, 7 out]
        n183 = local write "Status FTP move"(w398) -> ()
        n184 = case shown="False" w399 {
          tunnel: w398 -> [_ w411]
          tunnel: [errorcluster[][] [] ("ErrorArray") w410] -> w403
          tunnel: w404 -> [_ w409]
          tunnel: w401 -> [_ w408]
          tunnel: w402 -> [_ w407]
          tunnel: w400 -> [_ w406]
          frame False {
          }
          frame True {
            n185 = call "FTP Move files.vi"("File Management"=w408, "Unmanaged Files Queue"=w409, "FTP Creds"=w407, "File output directories"=w406, "Timing true or false to zip files"=w411) -> ("ErrorArray"=w410:errorcluster[][])  [unwired: 13 in, 1 out]
          }
        }
      }
      event "Manual FTP": Value Change {
        n186 = event-data() -> ()  [unwired: 1 in, 1 out]
        n187 = local write "Status FTP move"(TRUE ("Status FTP move")) -> ()
        n188 = call "FTP Move files.vi"("File Management"=w413, "Unmanaged Files Queue"=w415, "FTP Creds"=w414, "File output directories"=w412, "Timing true or false to zip files"=TRUE) -> ("ErrorArray"=w416:errorcluster[][])  [unwired: 13 in, 1 out]
      }
    }
    n189 = for {
      tunnel: w377 -> [w387]
      tunnel: w375 -> [w386] mode=indexing
      n190 = for {
        tunnel: w387 -> [w389]
        tunnel: w386 -> [w388] mode=indexing
        n191 = case shown="Error" w388 {
          selector: w388 -> [_ w393]
          tunnel: w389 -> [_ w397]
          frame No Error {
          }
          frame Error {
            n192 = Unbundle By Name(w393) -> ("source"=w392:string)
            n193 = Concatenate Strings("FTP Failed: " ("string"), w392) -> (w391:string)
            n194 = Bundle By Name(cluster=errorcluster {"status"=FALSE, "code"=0, "source"=""} ("error constant"), "status"=TRUE, "source"=w391) -> (w395:errorcluster)
            n195 = Enqueue Element(queue=w397, element=w395) -> ()  [unwired: 2 in, 3 out]
          }
        }
      }
    }
    n196 = call "Action Engine Shutdown.vi"("Shutdown"=enum16{"Write", "Read"}."Read") -> ("Shutdown"=w379:bool)  [unwired: 9 in, 1 out]
    "Status FTP move" <- FALSE ("Status FTP move")
  }
  n197 = while "FTP vs Local File size checks" {
    tunnel: w30 -> [w422]
    tunnel: w29 -> [w425]
    stop <- w420 stop-if-true
    n198 = local read "File Management"() -> (w427:T3)
    n199 = local read "File output directories"() -> (w424:T4)
    n200 = local read "FTP Creds"() -> (w423:T2)
    n201 = Wait (ms)(milliseconds to wait=u32 200) -> ()  [unwired: 1 out]
    n202 = Unbundle By Name(w427) -> ("Comp File Size"=w426:bool)
    n203 = case shown="False" w426 {
      tunnel: w427 -> [_ w432]
      tunnel: w425 -> [_ w431]
      tunnel: w424 -> [_ w430]
      tunnel: w423 -> [_ w429]
      tunnel: w422 -> [_ w428]
      frame False {
      }
      frame True {
        n204 = for {
          N: 1 -> [_]
          tunnel: [w438] -> w434
          shift-right: [w436] -> _
          shift-left: _ -> [w435]
          n205 = call "True at one time of day.vi"("Next start time in"=w435, "Time stamp from INI (only will use time Not date)"="Time DaY") -> ("next start time out"=w436:dbl, "Time Until Next Scan (H)"=→"Elapsed Time (H)":dbl, "Time has Elapsed"=w438:bool)  [unwired: 6 in, 1 out]
        }
        n206 = case shown="True" w434 {
          tunnel: w432 -> [_ w447]
          tunnel: w431 -> [_ w446]
          tunnel: w430 -> [_ w445]
          tunnel: w429 -> [_ w444]
          tunnel: w428 -> [_ w441]
          frame False {
          }
          frame True {
            w452 = "\r\n"
            n207 = call "Compare file to FTP directory.vi"("File Management"=w447, "FTP Creds"=w444, "File output directories"=w445, "Unmanaged Files Queue"=w446) -> ("number of unmached files"=w449:i32, "unmatched file names"=w448:string, "ErrorArray"=w440:errorcluster[][])  [unwired: 12 in, 1 out]
            n208 = local read "SITE ID"() -> (w450:string)
            n209 = Concatenate Strings("FTP VS DIR File sizes are different: " ("string"), w450) -> (w451:string)
            n210 = Greater Than 0?(x=w449) -> (x > 0?=w443:bool)
            n211 = Concatenate Strings(w451, w452, "These files have been re-queued for FTP move agian, check to make sure files are up to date and moving correctly.\nFiles of issue are listed below.\n\nLIST:" ("string"), w452, w448) -> (w442:string)
            n212 = for {
              tunnel: w441 -> [w456]
              tunnel: w440 -> [w455] mode=indexing
              n213 = for {
                tunnel: w456 -> [w458]
                tunnel: w455 -> [w457] mode=indexing
                n214 = case shown="Error" w457 {
                  selector: w457 -> [_ w461]
                  tunnel: w458 -> [_ w466]
                  frame No Error {
                  }
                  frame Error {
                    n215 = Unbundle By Name(w461) -> ("source"=w460:string)
                    n216 = Concatenate Strings("FTP Local File Compare Failed: " ("string"), w460) -> (w462:string)
                    n217 = Bundle By Name(cluster=errorcluster {"status"=FALSE, "code"=0, "source"=""} ("error constant"), "status"=TRUE, "source"=w462) -> (w464:errorcluster)
                    n218 = Enqueue Element(queue=w466, element=w464) -> ()  [unwired: 2 in, 3 out]
                  }
                }
              }
            }
            n219 = case shown="True" w443 {
              tunnel: w441 -> [_ w471]
              tunnel: w442 -> [_ w467]
              frame False {
              }
              frame True {
                n220 = Bundle By Name(cluster=errorcluster {"status"=FALSE, "code"=0, "source"=""} ("error constant"), "status"=TRUE, "source"=w467) -> (w469:errorcluster)
                n221 = Enqueue Element(queue=w471, element=w469) -> ()  [unwired: 2 in, 3 out]
              }
            }
          }
        }
      }
    }
    n222 = call "Action Engine Shutdown.vi"("Shutdown"=enum16{"Write", "Read"}."Read") -> ("Shutdown"=w420:bool)  [unwired: 9 in, 1 out]
  }
  n223 = flat-sequence {
    tunnel: w28 -> [w474]
    tunnel: [w473] -> w27
    tunnel: w7 -> [w472]
    tunnel: [w472] -> w4
    frame #0 {
      n224 = local read "Email Notification Cluster"() -> (w478:T5)
      n225 = local read "File output directories"() -> (w483:T4)
      n226 = local read "Addresses to Ping"() -> (w476:T1)
      n227 = local read "File Management"() -> (w485:T3)
      n228 = local read "Auto Archive"() -> (w481:bool)
      n229 = local read "FTP Creds"() -> (w480:T2)
      n230 = local read "recipients"() -> (w477:string[])
      n231 = local read "Time DaY"() -> (w484:timestamp)
      n232 = local read "Auto FTP"() -> (w482:bool)
      n233 = local read "SITE ID"() -> (w486:string)
      n234 = local read "hours"() -> (w479:u8)
      n235 = Bundle By Name(cluster=T8 {"Site ID"="", "File Management cluster"={"Comp File Size"=FALSE, "File Handle Method"=enum."Archive and zip in place from file *.ext list", "file extention list"=[]}, "time stamp"=timestamp(0 s since 1904-01-01), "File output directories"={"Archive Location"=path "", "Archive Location 2"=path "<Not A Path>", "OutPut Path"=path "", "Directory(s) To Scan Files"=[]}, "Auto FTP"=FALSE, "Auto Archive"=FALSE, "FTP CRED Cluster"={"Host"="", "UserName"="", "PassWord"="", "FTP File Path"="", "Timeout (S)"=60, "ActivePasive"=FALSE, "Binary Ascii"=FALSE, "Remote Port"=0}, "hours old date mod(hours)"=2, "Email Notification Cluster"={"Mail Server"="", "Return Address"="", "Email User Name"="", "Password"=""}, "Email Recipiant List"=[], "Addresses to Ping"=[]} ("Settings To Bini"), "Site ID"=w486, "File Management cluster"=w485, "time stamp"=w484, "File output directories"=w483, "Auto FTP"=w482, "Auto Archive"=w481, "FTP CRED Cluster"=w480, "hours old date mod(hours)"=w479, "Email Notification Cluster"=w478, "Email Recipiant List"=w477, "Addresses to Ping"=w476) -> (w487:T8)
      n236 = call "Bini output cluster ArchiveAndFtp.vi"("Settings To Bini"=w487) -> ("Bini Error out"=w475:errorcluster)  [unwired: 14 in]
      n237 = case shown="No Error" w475 {
        selector: w475 -> [_ w491]
        tunnel: w474 -> [w489 w492]
        tunnel: [w489 w490] -> w473
        frame No Error {
        }
        frame Error {
          n238 = Enqueue Element(queue=w492, element=w491) -> (queue out=w490:refnum<queue>)  [unwired: 2 in, 2 out]
        }
      }
    }
  }
  n239 = Get Queue Status(queue=w27, return elements? (F)=TRUE) -> (queue out=w20:refnum<queue>, error out=w19:errorcluster, elements=w25:errorcluster[])  [unwired: 1 in, 5 out]
  n240 = for {
    tunnel: w25 -> [w494] mode=indexing
    tunnel: [w493] -> w24 mode=indexing
    n241 = Unbundle By Name(w494) -> ("source"=w493:string)
  }
  n242 = Flush Queue(queue=w20, error in (no error)=w19) -> (queue out=w22:refnum<queue>, error out=w21:errorcluster)  [unwired: 1 out]
  n243 = Release Queue(queue=w22, error in (no error)=w21) -> (error out=w5:errorcluster)  [unwired: 1 in, 2 out]
  n244 = Flush Queue(queue=w4, error in (no error)=w5) -> (queue out=w6:refnum<queue>, error out=w3:errorcluster)  [unwired: 1 out]
  n245 = Release Queue(queue=w6, error in (no error)=w3) -> (error out=w2:errorcluster)  [unwired: 1 in, 2 out]
  n246 = Array To Spreadsheet String(array=w24, 3:"%s" ("format string")) -> (spreadsheet string=w8:string)  [unwired: 1 in]
  n247 = call <vilib>:"Application Directory.vi"() -> ("Application Directory"=w17:path)
  n248 = Build Path(base path=w17, name or relative path="File Archive and FTP Error.LOG") -> (appended path=w14:path)
  n249 = Open/Create/Replace File(file path (use dialog)=w14, error in=w2, operation (0:open)=T6."replace or create", access (0:read/write)=enum16{"read/write", "read-only", "write-only"}."read-only") -> (refnum out=w15:refnum<file>, error out=w16:errorcluster)  [unwired: 2 in, 1 out]
  n250 = Write to Text File(file (use dialog)=w15, text=w8, error in=w16) -> (refnum out=w11:refnum<file>, error out=w10:errorcluster)  [unwired: 1 in, 1 out]
  n251 = control-ref of="This Application"() -> (w1:refnum<vi>)
  n252 = Close File(refnum=w11, error in=w10) -> (error out=w9:errorcluster)  [unwired: 1 out]
  n253 = call <vilib>:"Clear Errors.vi"("error in (no error)"=w9) -> ("error out"=w33:errorcluster)  [unwired: 6 in]
  n254 = property class="App"(reference=w1, error in=w33) -> (error out=w34:errorcluster, "App.Kind"=w35:T12)  [unwired: 1 out]
  n255 = case shown="\"Run Time System\"" w35 {
    tunnel: w34 -> [_ _ _ _ _ _ _]
    frame "invalid app kind", Default {
    }
    frame "Development System" {
      w496 = T13 5 items=["User Home"=0, "User Desktop"=1, "User Documents"=2, "User Application Data"=3, "User Preferences"=4, "User Temporary"=5, "Public Documents"=6, "Public Application Data"=7, "Public Preferences"=8, "Public Cache"=13, "System Core Libraries"=9, "System Installed Libraries"=10, "Application Files"=11, "Boot Volume Root"=12] ("system directory type")
      n256 = call <vilib>:"Get System Directory.vi"("create directory if not found? (F)"=TRUE, "system directory type"=w496) -> ("system directory"=w498:path)  [unwired: 9 in]
      n257 = Build Path(base path=w498, name or relative path="Archive and ftp") -> (appended path=w500:path)
      n258 = Delete(path (use dialog)=w500, entire hierarchy (F)=TRUE) -> (error out=w495:errorcluster)  [unwired: 3 in, 2 out]
      n259 = call <vilib>:"Clear Errors.vi"("error in (no error)"=w495) -> ()  [unwired: 6 in, 1 out]
    }
    frame "Run Time System" {
      n260 = flat-sequence {
        frame #0 {
          w503 = T13 5 items=["User Home"=0, "User Desktop"=1, "User Documents"=2, "User Application Data"=3, "User Preferences"=4, "User Temporary"=5, "Public Documents"=6, "Public Application Data"=7, "Public Preferences"=8, "Public Cache"=13, "System Core Libraries"=9, "System Installed Libraries"=10, "Application Files"=11, "Boot Volume Root"=12] ("system directory type")
          n261 = call <vilib>:"Get System Directory.vi"("create directory if not found? (F)"=TRUE, "system directory type"=w503) -> ("system directory"=w505:path)  [unwired: 9 in]
          n262 = Build Path(base path=w505, name or relative path="Archive and ftp") -> (appended path=w507:path)
          n263 = Delete(path (use dialog)=w507, entire hierarchy (F)=TRUE) -> (error out=w502:errorcluster)  [unwired: 3 in, 2 out]
          n264 = call <vilib>:"Clear Errors.vi"("error in (no error)"=w502) -> ()  [unwired: 6 in, 1 out]
        }
        frame #1 {
          n265 = Quit LabVIEW() -> ()  [unwired: 1 in]
        }
      }
    }
    frame "Student Edition" {
    }
    frame "Embedded LabVIEW" {
    }
    frame "Evaluation" {
    }
    frame "Custom" {
    }
  }
